vi "read_data.vi"(8 "Error_IN":errorcluster caption="error out", 9 "Notifier_IN":refnum<notifier>, 10 "Q_Data_Err_IN":errorcluster caption="에러 입력", 11 "Q_Data_IN":refnum<queue>) -> (2 "Q_Data_Err_OUT":errorcluster caption="에러 출력", 3 "Q_Data_OUT":refnum<queue>)   [LabVIEW 2019]
uses:
  <vilib>/Platform/TimedLoop/XDataNode/timing_clust.ctl
  <vilib>/Platform/TimedLoop/XDataNode/nitl_modes.ctl
  <vilib>/Platform/TimedLoop/XDataNode/wakeup.ctl
  <vilib>/Platform/TimedLoop/XDataNode/XDataNode.xnode
  <vilib>/Platform/TimedLoop/XDataNode/XDNodeRunTimeDep.lvlib
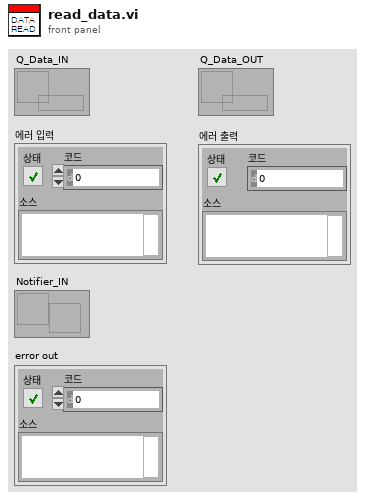
[diagram p1: front panel]
types:
  T1 = typedef "XDNodeRunTimeDep.lvlib/timing_clust.ctl" = cluster{"Expected End [f-1]":u64, "Actual End [f-1]":u64, "Finished Late? [f-1]":bool, "Expected End [i-1]":u64, "Actual End [i-1]":u64, "Finished Late? [i-1]":bool, "Expected Start [i]":u64, "Actual Start [i]":u64, "Expected Start [f]":u64, "Actual Start [f]":u64, "Source Name":string, "Structure Name":string, "Period":i64, "Deadline":i64, "Offset":i64, "Start":i64, "Priority":i32, "Timeout":i32, "Mode":T2, "Wakeup Reason":T3, "Error":errorcluster, "Source Type":string, "Secondary Source Type":string, "Global End Time":u64, "Global Start Time":u64, "Frame Duration":u64, "Iteration Duration":u64, "Assigned CPU":i32, "I/O Scan Engine Mode":u32}
  T2 = typedef "XDNodeRunTimeDep.lvlib/nitl_modes.ctl" = enum32{"No Change", "Process missed periods, maintain original phase", "Discard missed periods, maintain original phase", "Process missed periods, ignore original phase", "Discard missed periods, ignore original phase"}
  T3 = typedef "XDNodeRunTimeDep.lvlib/wakeup.ctl" = enum32{"Normal", "Aborted", "Asynchronous wakeup", "Timing source error", "Timed loop error", "Timeout"}
  T4 = cluster{"FPGA_Data":sgl[], "Tick":u32, "Cmd":string, "Param":variant}
  T5 = typedef "CANFrameControl.ctl" = cluster{"identifier":u32, "extended?":bool, "type":u8, "payload":u8[]}
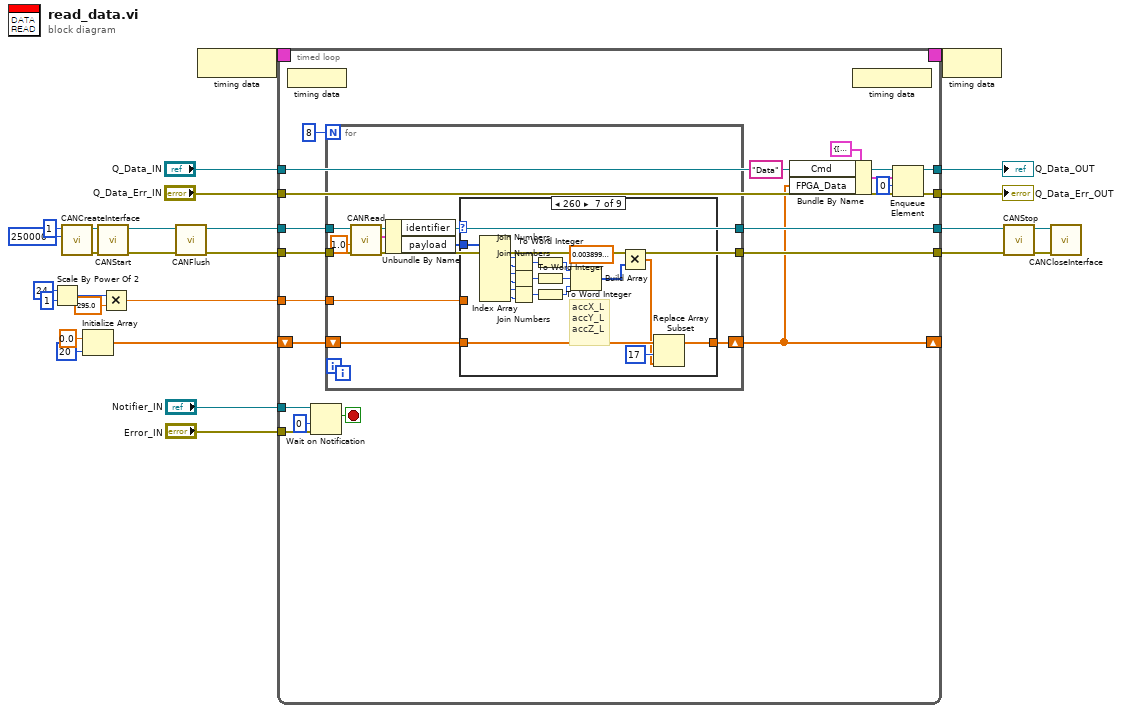
[diagram p0: block diagram]
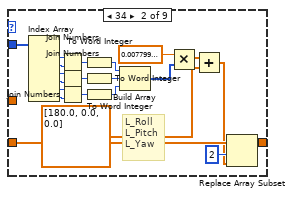
[diagram p3: hidden frame]
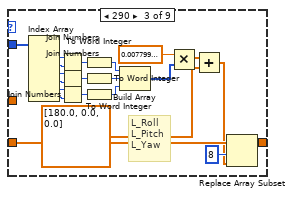
[diagram p4: hidden frame]
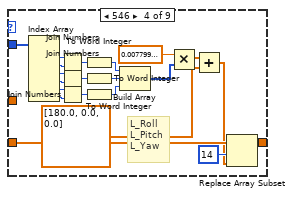
[diagram p5: hidden frame]
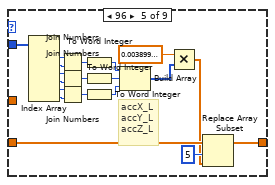
[diagram p6: hidden frame]
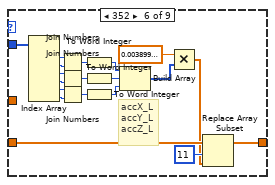
[diagram p7: hidden frame]
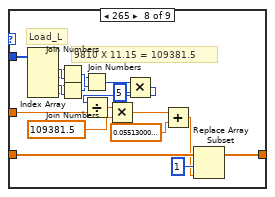
[diagram p8: hidden frame]
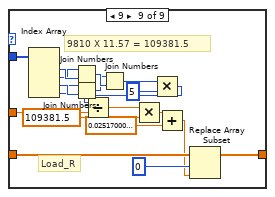
[diagram p9: hidden frame]
diagram:
  n1 = Scale By Power Of 2(n=i16 24, x=u32 1) -> (x*2^n=w17:u32)
  n2 = call <vilib>:"CANCreateInterface.vi"("baud rate (125000 bps)"=u32 250000, "interface index"=u32 1) -> ("error out"=w25:errorcluster, "interface object out"=w26:refnum<k20>)  [unwired: 8 in]
  n3 = Initialize Array(sgl 0.0 ("timeout (0 s)"), 20 ("차원 크기")) -> (w18:sgl[])
  n4 = call <vilib>:"CANStart.vi"("error in (no error)"=w25, "interface object in"=w26) -> ("error out"=w3:errorcluster, "interface object out"=w4:refnum<k20>)  [unwired: 8 in]
  n5 = Multiply ("곱하기")(x=w17, y=295.0) -> (x*y=w13:dbl)
  n6 = call <vilib>:"CANFlush.vi"("error in (no error)"=w3, "interface object in"=w4) -> ("error out"=w1:errorcluster, "interface object out"=w2:refnum<k20>)  [unwired: 8 in]
  n7 = node-c288() -> (w12:T1)
  n8 = timed-loop {
    tunnel: w2 -> [w48]
    tunnel: w1 -> [w47]
    tunnel: [w46] -> w22
    tunnel: [w43] -> w21
    shift-right: [w37] -> _
    shift-left: w18 -> [w45]
    tunnel: w13 -> [w44]
    timing: w12 -> [_]
    timing-out: [_] -> w11
    tunnel: "Q_Data_IN" -> [w40]
    tunnel: "Q_Data_Err_IN" -> [w39]
    tunnel: [w34] -> w8
    tunnel: [w33] -> w7
    tunnel: "Notifier_IN" -> [w30]
    tunnel: "Error_IN" -> [w29]
    stop <- w31 stop-if-true
    n9 = node-c288() -> ()  [unwired: 1 in]
    n10 = Wait on Notification(notifier=w30, timeout in ms (-1)=0 ("타임아웃(ms) (-1)"), error in (no error)=w29) -> (notification=w31:bool)  [unwired: 1 in, 3 out]
    n11 = for {
      N: 8 -> [_]
      tunnel: w44 -> [w54]
      shift-right: [w49] -> w37
      shift-left: w45 -> [w55]
      tunnel: w47 -> [w58]
      tunnel: [w51] -> w43
      tunnel: w48 -> [w59]
      tunnel: [w57] -> w46
      n12 = call <vilib>:"CANRead.vi"("error in (no error)"=w58, "timeout (0 s)"=1.0, "interface object in"=w59) -> ("error out"=w51:errorcluster, "CAN frame"=w56:T5, "interface object out"=w57:refnum<k20>)  [unwired: 5 in, 1 out]
      n13 = Unbundle By Name(w56) -> ("identifier"=w53:u32, "payload"=w52:u8[])
      n14 = case shown="260" w53 {
        tunnel: w52 -> [_ w75 w96 w117 w136 w155 w174 w190 w206]
        tunnel: w55 -> [w60 w74 w95 w116 w135 w154 w173 w199 w218]
        tunnel: [w60 w72 w93 w114 w133 w152 w171 w197 w216] -> w49
        tunnel: w54 -> [_ _ _ _ _ _ _ w187 w207]
        frame 0, Default {
        }
        frame 34 {
          # "L_Roll\nL_Pitch\nL_Yaw"
          n15 = Index Array(array=w75) -> (element #1=w76:u8, element #2=w77:u8, element #3=w78:u8, element #4=w79:u8, element #5=w80:u8, element #6=w81:u8)  [unwired: 6 in]
          n16 = Join Numbers(hi=w76, lo=w77) -> ((hi.lo)=w70:u16)
          n17 = Join Numbers(hi=w78, lo=w79) -> ((hi.lo)=w68:u16)
          n18 = Join Numbers(hi=w80, lo=w81) -> ((hi.lo)=w69:u16)
          n19 = To Word Integer(number=w70) -> (16bit integer=w66:i16)
          n20 = To Word Integer(number=w68) -> (16bit integer=w65:i16)
          n21 = To Word Integer(number=w69) -> (16bit integer=w64:i16)
          n22 = Build Array(w66, w65, w64) -> (w63:i16[])
          n23 = Multiply ("곱하기")(x=sgl 0.0078, y=w63) -> (x*y=w62:sgl[])
          n24 = Add(x=w62, y=sgl[] [180.0, 0.0, 0.0]) -> (x+y=w71:sgl[])
          n25 = Replace Array Subset(array=w74, new element=w71, index=2 ("인덱스")) -> (w72:sgl[])
        }
        frame 290 {
          # "L_Roll\nL_Pitch\nL_Yaw"
          n26 = Index Array(array=w96) -> (element #1=w97:u8, element #2=w98:u8, element #3=w99:u8, element #4=w100:u8, element #5=w101:u8, element #6=w102:u8)  [unwired: 6 in]
          n27 = Join Numbers(hi=w97, lo=w98) -> ((hi.lo)=w91:u16)
          n28 = Join Numbers(hi=w99, lo=w100) -> ((hi.lo)=w89:u16)
          n29 = Join Numbers(hi=w101, lo=w102) -> ((hi.lo)=w90:u16)
          n30 = To Word Integer(number=w91) -> (16bit integer=w87:i16)
          n31 = To Word Integer(number=w89) -> (16bit integer=w86:i16)
          n32 = To Word Integer(number=w90) -> (16bit integer=w85:i16)
          n33 = Build Array(w87, w86, w85) -> (w84:i16[])
          n34 = Multiply ("곱하기")(x=sgl 0.0078, y=w84) -> (x*y=w83:sgl[])
          n35 = Add(x=w83, y=sgl[] [180.0, 0.0, 0.0]) -> (x+y=w92:sgl[])
          n36 = Replace Array Subset(array=w95, new element=w92, index=8 ("인덱스")) -> (w93:sgl[])
        }
        frame 546 {
          # "L_Roll\nL_Pitch\nL_Yaw"
          n37 = Index Array(array=w117) -> (element #1=w118:u8, element #2=w119:u8, element #3=w120:u8, element #4=w121:u8, element #5=w122:u8, element #6=w123:u8)  [unwired: 6 in]
          n38 = Join Numbers(hi=w118, lo=w119) -> ((hi.lo)=w112:u16)
          n39 = Join Numbers(hi=w120, lo=w121) -> ((hi.lo)=w110:u16)
          n40 = Join Numbers(hi=w122, lo=w123) -> ((hi.lo)=w111:u16)
          n41 = To Word Integer(number=w112) -> (16bit integer=w108:i16)
          n42 = To Word Integer(number=w110) -> (16bit integer=w107:i16)
          n43 = To Word Integer(number=w111) -> (16bit integer=w106:i16)
          n44 = Build Array(w108, w107, w106) -> (w105:i16[])
          n45 = Multiply ("곱하기")(x=sgl 0.0078, y=w105) -> (x*y=w104:sgl[])
          n46 = Add(x=w104, y=sgl[] [180.0, 0.0, 0.0]) -> (x+y=w113:sgl[])
          n47 = Replace Array Subset(array=w116, new element=w113, index=14 ("인덱스")) -> (w114:sgl[])
        }
        frame 96 {
          # "accX_L\naccY_L\naccZ_L"
          n48 = Index Array(array=w136) -> (element #1=w137:u8, element #2=w138:u8, element #3=w139:u8, element #4=w140:u8, element #5=w141:u8, element #6=w142:u8)  [unwired: 6 in]
          n49 = Join Numbers(hi=w137, lo=w138) -> ((hi.lo)=w132:u16)
          n50 = Join Numbers(hi=w139, lo=w140) -> ((hi.lo)=w130:u16)
          n51 = Join Numbers(hi=w141, lo=w142) -> ((hi.lo)=w131:u16)
          n52 = To Word Integer(number=w132) -> (16bit integer=w128:i16)
          n53 = To Word Integer(number=w130) -> (16bit integer=w127:i16)
          n54 = To Word Integer(number=w131) -> (16bit integer=w126:i16)
          n55 = Build Array(w128, w127, w126) -> (w125:i16[])
          n56 = Multiply ("곱하기")(x=sgl 0.0039, y=w125) -> (x*y=w124:sgl[])
          n57 = Replace Array Subset(array=w135, new element=w124, index=5 ("인덱스")) -> (w133:sgl[])
        }
        frame 352 {
          # "accX_L\naccY_L\naccZ_L"
          n58 = Index Array(array=w155) -> (element #1=w156:u8, element #2=w157:u8, element #3=w158:u8, element #4=w159:u8, element #5=w160:u8, element #6=w161:u8)  [unwired: 6 in]
          n59 = Join Numbers(hi=w156, lo=w157) -> ((hi.lo)=w151:u16)
          n60 = Join Numbers(hi=w158, lo=w159) -> ((hi.lo)=w149:u16)
          n61 = Join Numbers(hi=w160, lo=w161) -> ((hi.lo)=w150:u16)
          n62 = To Word Integer(number=w151) -> (16bit integer=w147:i16)
          n63 = To Word Integer(number=w149) -> (16bit integer=w146:i16)
          n64 = To Word Integer(number=w150) -> (16bit integer=w145:i16)
          n65 = Build Array(w147, w146, w145) -> (w144:i16[])
          n66 = Multiply ("곱하기")(x=sgl 0.0039, y=w144) -> (x*y=w143:sgl[])
          n67 = Replace Array Subset(array=w154, new element=w143, index=11 ("인덱스")) -> (w152:sgl[])
        }
        frame 608 {
          # "accX_L\naccY_L\naccZ_L"
          n68 = Index Array(array=w174) -> (element #1=w175:u8, element #2=w176:u8, element #3=w177:u8, element #4=w178:u8, element #5=w179:u8, element #6=w180:u8)  [unwired: 6 in]
          n69 = Join Numbers(hi=w175, lo=w176) -> ((hi.lo)=w170:u16)
          n70 = Join Numbers(hi=w177, lo=w178) -> ((hi.lo)=w168:u16)
          n71 = Join Numbers(hi=w179, lo=w180) -> ((hi.lo)=w169:u16)
          n72 = To Word Integer(number=w170) -> (16bit integer=w166:i16)
          n73 = To Word Integer(number=w168) -> (16bit integer=w165:i16)
          n74 = To Word Integer(number=w169) -> (16bit integer=w164:i16)
          n75 = Build Array(w166, w165, w164) -> (w163:i16[])
          n76 = Multiply ("곱하기")(x=sgl 0.0039, y=w163) -> (x*y=w162:sgl[])
          n77 = Replace Array Subset(array=w173, new element=w162, index=17 ("인덱스")) -> (w171:sgl[])
        }
        frame 265 {
          # "9810 X 11.15 = 109381.5"
          # "Load_L"
          n78 = Index Array(array=w190) -> (element #1=w196:u8, element #2=w195:u8, element #3=w194:u8, element #4=w193:u8)  [unwired: 4 in]
          n79 = Join Numbers(hi=w195, lo=w196) -> ((hi.lo)=w192:u16)
          n80 = Join Numbers(hi=w193, lo=w194) -> ((hi.lo)=w191:u16)
          n81 = Join Numbers(hi=w191, lo=w192) -> ((hi.lo)=w181:u32)
          n82 = Multiply ("곱하기")(x=w181, y=u32 5) -> (x*y=w188:u32)
          n83 = Divide ("나누기")(x=w188, y=w187) -> (x/y=w186:dbl)
          n84 = Multiply ("곱하기")(x=w186, y=109381.5) -> (x*y=w182:dbl)
          n85 = Add ("더하기")(x=w182, y=0.0551300011575222) -> (x+y=w183:sgl)
          n86 = Replace Array Subset(array=w199, new element=w183, index=1 ("인덱스")) -> (w197:sgl[])
        }
        frame 9 {
          # "9810 X 11.57 = 109381.5"
          # "Load_R"
          n87 = Index Array(array=w206) -> (element #1=w215:u8, element #2=w214:u8, element #3=w213:u8, element #4=w212:u8)  [unwired: 4 in]
          n88 = Join Numbers(hi=w214, lo=w215) -> ((hi.lo)=w211:u16)
          n89 = Join Numbers(hi=w212, lo=w213) -> ((hi.lo)=w210:u16)
          n90 = Join Numbers(hi=w210, lo=w211) -> ((hi.lo)=w200:u32)
          n91 = Multiply(x=w200, y=u32 5) -> (x*y=w208:u32)
          n92 = Divide ("나누기")(x=w208, y=w207) -> (x/y=w201:dbl)
          n93 = Multiply ("곱하기")(x=w201, y=109381.5) -> (x*y=w204:dbl)
          n94 = Add ("더하기")(x=w204, y=0.02517000027000904) -> (x+y=w202:sgl)
          n95 = Replace Array Subset(array=w218, new element=w202, index=0 ("인덱스")) -> (w216:sgl[])
        }
      }
    }
    n96 = Bundle By Name(cluster=T4 {"FPGA_Data"=[], "Tick"=0, "Cmd"="", "Param"=variant} ("원소"), "Cmd"="Data", "FPGA_Data"=w37) -> (w36:T4)
    n97 = node-c288() -> ()  [unwired: 1 out]
    n98 = Enqueue Element(queue=w40, element=w36, timeout in ms (-1)=0 ("타임아웃(ms) (-1)"), error in (no error)=w39) -> (queue out=w34:refnum<queue>, error out=w33:errorcluster)  [unwired: 1 out]
  }
  "Q_Data_OUT" <- w8
  "Q_Data_Err_OUT" <- w7
  n99 = node-c288(w11) -> ()
  n100 = call <vilib>:"CANStop.vi"("error in (no error)"=w21, "interface object in"=w22) -> ("error out"=w24:errorcluster, "interface object out"=w23:refnum<k20>)  [unwired: 8 in]
  n101 = call <vilib>:"CANCloseInterface.vi"("error in (no error)"=w24, "interface object in"=w23) -> ()  [unwired: 9 in, 1 out]
